vi "regUserEvents.vi"(8 "error in (no error)":errorcluster, 11 "TcpServer.lvclass":refnum<class "TcpServer.lvclass">) -> (0 "error out":errorcluster, 3 "TcpServer.lvclass":refnum<class "TcpServer.lvclass">)   [LabVIEW 2018, in "TcpServer.lvclass"]
uses:
  TcpServer.lvclass
  userEventTypeDef.ctl
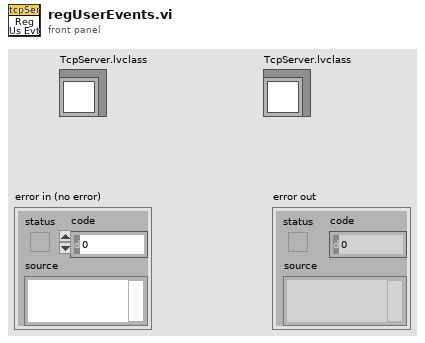
[diagram p1: front panel]
types:
  T1 = typedef "TcpServer.lvclass/userEventTypeDef.ctl" = cluster{"CmdRead":refnum<user-event>, "EvtRead":refnum<user-event>, "GenRead":refnum<user-event>, "ConnStatus":refnum<user-event>}
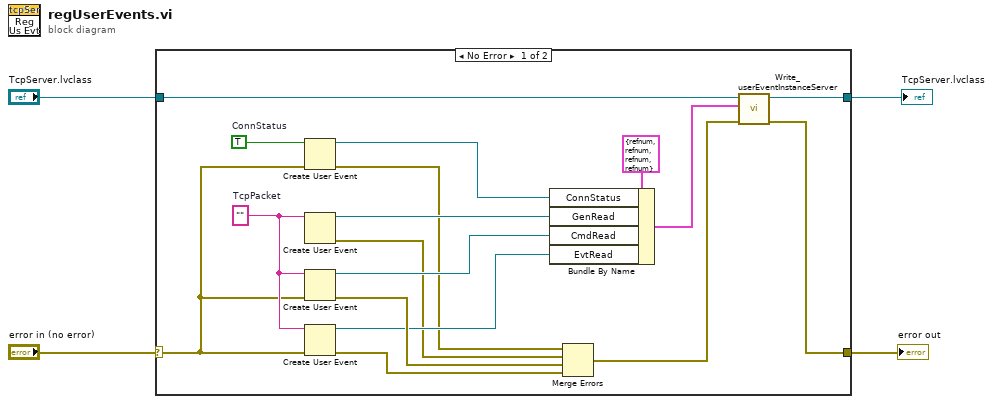
[diagram p0: block diagram]
diagram:
  n1 = case shown="No Error" "error in (no error)" {
    selector: "error in (no error)" -> [w7 w23]
    tunnel: [w12 w23] -> w3
    tunnel: [w13 w22] -> w1
    tunnel: "TcpServer.lvclass" -> [w14 w22]
    frame No Error {
      w9 = TRUE  # ConnStatus
      w11 = ""  # TcpPacket
      n2 = Create User Event(user event datatype=w9, error in=w7) -> (user event=w8:refnum<user-event>, error out=w5:errorcluster)
      n3 = Create User Event(user event datatype=w11) -> (user event=w10:refnum<user-event>, error out=w6:errorcluster)  [unwired: 1 in]
      n4 = Create User Event(user event datatype=w11, error in=w7) -> (user event=w17:refnum<user-event>, error out=w19:errorcluster)
      n5 = Create User Event(user event datatype=w11, error in=w7) -> (user event=w15:refnum<user-event>, error out=w16:errorcluster)
      n6 = Bundle By Name(cluster=T1 {"CmdRead"=refnum, "EvtRead"=refnum, "GenRead"=refnum, "ConnStatus"=refnum} ("userEventInstancesCmd"), "ConnStatus"=w8, "GenRead"=w10, "CmdRead"=w17, "EvtRead"=w15) -> (w21:T1)
      n7 = Merge Errors(w5, w6, w19, w16) -> (w20:errorcluster)
      n8 = call-dynamic "Write_userEventInstanceServer.vi"("error in (no error)"=w20, "userEventInstanceServer"=w21, "TcpServer in"=w14) -> ("error out"=w12:errorcluster, "TcpServer out"=w13:refnum<class "TcpServer.lvclass">)  [unwired: 7 in]
    }
    frame Error {
    }
  }
  "error out" <- w3
  "TcpServer.lvclass" <- w1
